vi "Master on Desktop（RTU）.vi"() -> ()   [LabVIEW 2017]
doc: "Demonstrates how to use Modbus functions to create a master communicating with a Modbus slave. It shows an interactive UI to allow users manually read and write the coils on the slave using TCP connection. Users can also change the timeout for reading operation if the network state is not good."
uses:
  <vilib>/Modbus/subvis/Modbus API/Modbus API.lvclass/Modbus API.ctl
  <vilib>/Modbus/subvis/Transmission Data Unit (ADU)/Transmission Data Unit/Transmission Data Unit.lvclass/Transmission Data Unit.ctl
  <vilib>/Modbus/master/Data Access/Read Timeout/Set Read Timeout.vi
  <vilib>/Modbus/subvis/Modbus API/Read Transmission Data Unit.vi
  <vilib>/Modbus/subvis/Modbus API/Write Transmission Data Unit.vi
  <vilib>/Modbus/subvis/Transmission Data Unit (ADU)/Transmission Data Unit/Data Access/timeouts/Write read operation timeout.vi
  <vilib>/Modbus/master/Modbus Master.lvclass
  D:/Program Files (x86)/National Instruments/LabVIEW 2017/vi.lib/Modbus/subvis/Modbus API/Modbus API.lvclass
  <vilib>/Modbus/master/Create Master Instance (Serial).vi
  <vilib>/Modbus/subvis/Transmission Data Unit (ADU)/Transmission Data Unit/Transmission Data Unit.lvclass
panel:
  in  "VISA resource name":refnum<visa-resource-name>
  in  "baud rate (9600)":u32=9600
  in  "Set Read Timeout":bool
  in  "Read Timeout (ms)":i32=5000
  in  "Read Count":u16=10
  in  "Stop":bool
  in  "Read":bool
  out "Coil Values Read":bool[](array[boolean])
  in  "Write":bool
  in  "Coil Values to Write":bool[](array[boolean])
  # "Overview: Demonstrates the use of the Modbus Master VIs to create a Modbus master and use the Modbus master to read and write coil values on a Modbus slave.\nRequirements: LabVIEW Datalogging and Supervisory Control Module\nInstructions:\n1. Ensure Slave On Desktop.vi is already running.\n2. Run the VI.\n3. Click Stop to stop the VI."
  # "Write Operation"
  # "Read Operation"
  # "Set Timeout For Read Operation"
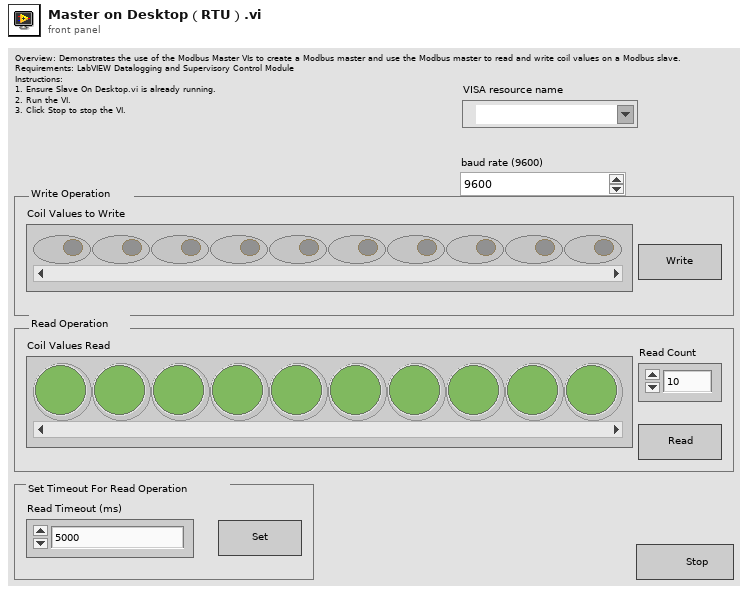
[diagram p1: front panel]
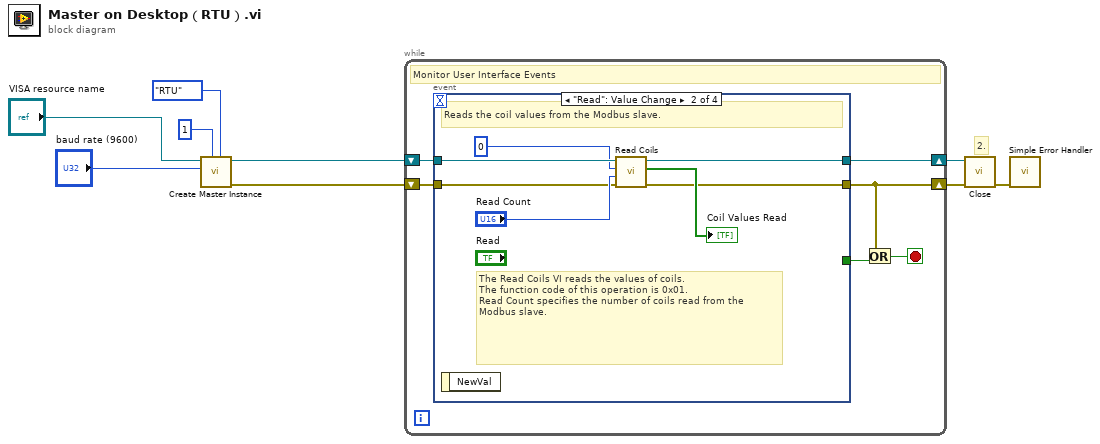
[diagram p0: block diagram]
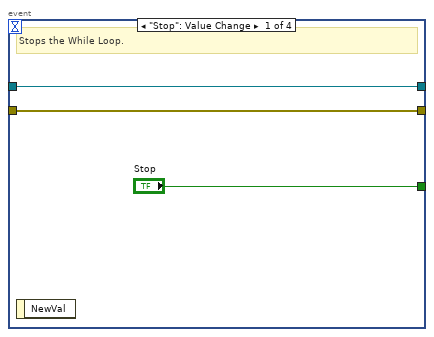
[diagram p2: hidden frame]
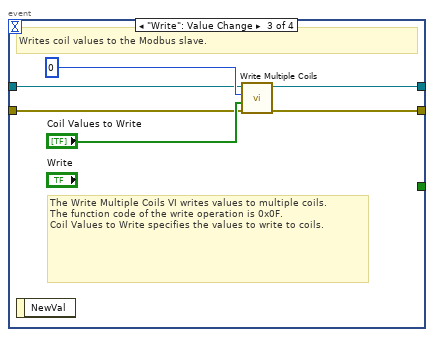
[diagram p3: hidden frame]
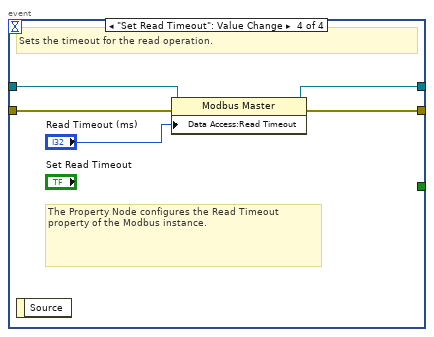
[diagram p4: hidden frame]
diagram:
  # "2."
  n1 = call-poly <vilib>:"Create Master Instance.vi"("serial type"=enum16{"RTU", "ASCII"}."RTU", "unit ID"=u8 1, "baud rate (9600)"="baud rate (9600)", "VISA resource name"="VISA resource name") -> ("error out"=w8:errorcluster, "serial master instance"=w9:refnum<class "Modbus Master.lvclass">)  [unwired: 6 in]
  n2 = while {
    shift-right: [w14] -> w6
    shift-left: w9 -> [w15]
    shift-right: [w12] -> w7
    shift-left: w8 -> [w13]
    stop <- w10 stop-if-true
    # "Monitor User Interface Events"
    n3 = event shown="[1] \"Read\": Value Change" {
      selector: _ -> [_ _ _ _]
      dyn-events: _ -> [_ _ _ _]
      timeout: _ -> [_ _ _ _]
      tunnel: ["Stop" _ _ _] -> w11
      tunnel: w15 -> [w17 w25 w29 w36]
      tunnel: [w17 w24 w28 w34] -> w14
      tunnel: w13 -> [w18 w20 w27 w35]
      tunnel: [w18 w19 w26 w33] -> w12
      event "Stop": Value Change {
        # "Stops the While Loop."
        n4 = event-data() -> ()  [unwired: 1 in, 1 out]
      }
      event "Read": Value Change {
        # "The Read Coils VI reads the values of coils.\nThe function code of this operation is 0x01.\nRead Count specifies the number of coils read from the Modbus slave."
        # "Reads the coil values from the Modbus slave."
        n5 = event-data() -> ()  [unwired: 1 in, 1 out]
        n6 = call-dynamic "Read Coils.vi"("error in (no error)"=w20, "number of coils"="Read Count", "starting address"=u16 0, "Modbus master in"=w25) -> ("error out"=w19:errorcluster, "coil values"=→"Coil Values Read":bool[], "Modbus master out"=w24:refnum<class "Modbus Master.lvclass">)  [unwired: 5 in]
      }
      event "Write": Value Change {
        # "The Write Multiple Coils VI writes values to multiple coils.\nThe function code of the write operation is 0x0F.\nCoil Values to Write specifies the values to write to coils."
        # "Writes coil values to the Modbus slave."
        n7 = event-data() -> ()  [unwired: 1 in, 1 out]
        n8 = call-dynamic "Write Multiple Coils.vi"("error in (no error)"=w27, "coil values"="Coil Values to Write", "starting address"=u16 0, "Modbus master in"=w29) -> ("error out"=w26:errorcluster, "Modbus master out"=w28:refnum<class "Modbus Master.lvclass">)  [unwired: 6 in]
      }
      event "Set Read Timeout": Value Change {
        # "The Property Node configures the Read Timeout property of the Modbus instance."
        # "Sets the timeout for the read operation."
        n9 = event-data() -> ()  [unwired: 1 in, 1 out]
        n10 = property class="Modbus Master"(reference=w36, error in=w35, "Data Access:Read Timeout"="Read Timeout (ms)") -> (reference out=w34:refnum<class "Modbus Master.lvclass">, error out=w33:errorcluster)
      }
    }
    n11 = Or(x=w12, y=w11) -> (x .or. y?=w10:bool)
  }
  n12 = call-dynamic "Close.vi"("error in (no error)"=w7, "Modbus master in"=w6) -> ("error out"=w5:errorcluster)  [unwired: 9 in]
  n13 = call <vilib>:"Simple Error Handler.vi"("error in (no error)"=w5) -> ()  [unwired: 4 in, 5 out]
